vi "Part 1.vi"(11 "Input":string) -> (3 "Output":i64)   [LabVIEW 2021]
uses:
  8e0448e5-4d13-43f9-9dbd-05e23abb9177.vi
  <userlib>/_OpenG.lib/string/string.llb/Convert EOLs (String)__ogtk.vi
panel:
  out "array":string[](array[string])
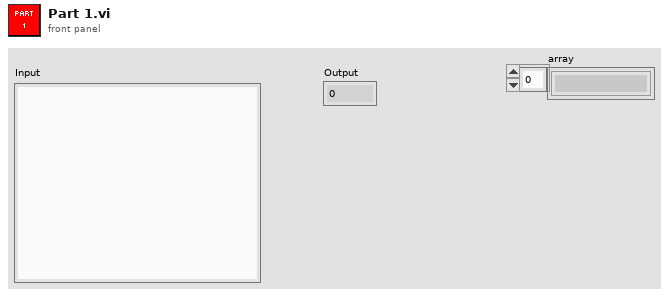
[diagram p1: front panel]
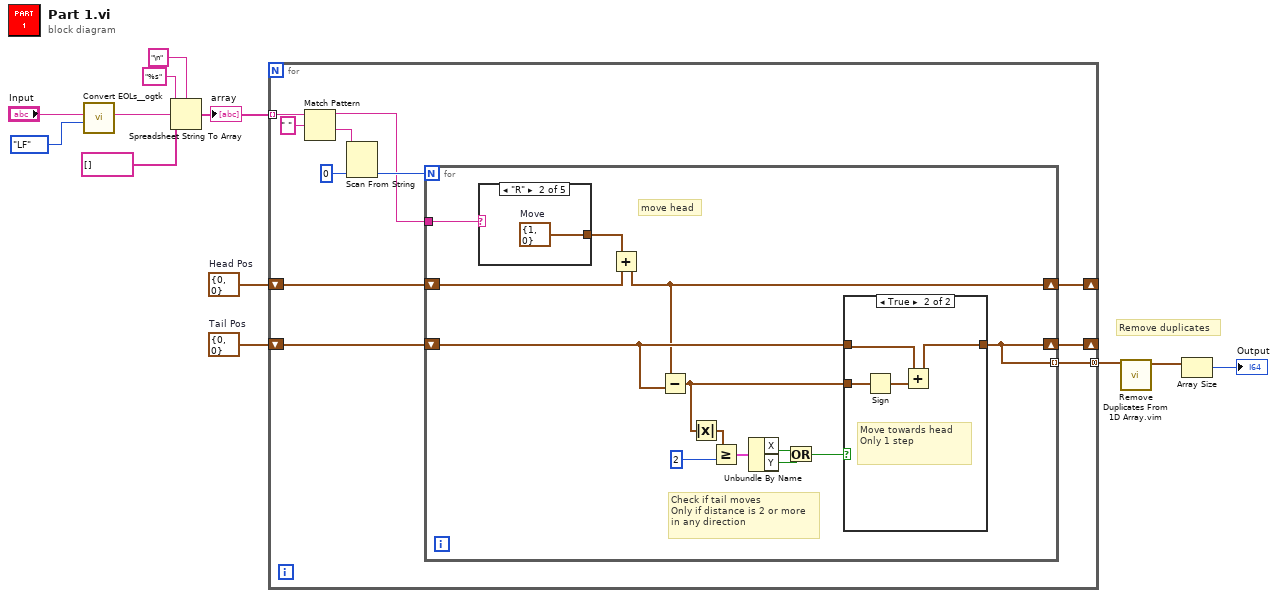
[diagram p0: block diagram]
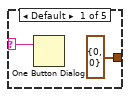
[diagram p3: hidden frame]
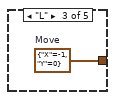
[diagram p4: hidden frame]
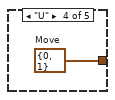
[diagram p5: hidden frame]
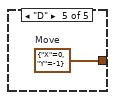
[diagram p6: hidden frame]
diagram:
  w4 = cluster{"X":i32, "Y":i32} {"X"=0, "Y"=0}  # Tail Pos
  w5 = cluster{"X":i32, "Y":i32} {"X"=0, "Y"=0}  # Head Pos
  # "Remove duplicates"
  n1 = call-poly <userlib>:"Convert EOLs__ogtk.vi"("Convert to:"=enum16{"CR", "LF", "CRLF"}."LF", "String in"="Input") -> ("String out"=w8:string)  [unwired: 9 in]
  n2 = Spreadsheet String To Array(delimiter (Tab)="\n", format string="%s", spreadsheet string=w8, array type (2D Dbl)=string[] []) -> (array=w6:string[])
  "array" <- w6
  n3 = for {
    tunnel: w6 -> [w23] mode=indexing
    shift-right: [w16] -> _
    shift-left: w5 -> [w18]
    shift-right: [w14] -> _
    shift-left: w4 -> [w17]
    tunnel: [w13] -> w3 mode=concatenating
    n4 = Match Pattern(string=w23, regular expression=" ") -> (before substring=w15:string, after substring=w21:string)  [unwired: 1 in, 2 out]
    n5 = Scan From String(input string=w21, default 1=0) -> (output 1=w19:i32)  [unwired: 3 in, 3 out]
    n6 = for {
      N: w19 -> [_]
      shift-right: [w25] -> w16
      shift-left: w18 -> [w35]
      shift-right: [w24] -> w14
      shift-left: w17 -> [w27]
      tunnel: w15 -> [w36]
      tunnel: [w24] -> w13 mode=indexing
      # "Check if tail moves\nOnly if distance is 2 or more\nin any direction"
      # "move head"
      n7 = case shown="\"R\"" w36 {
        selector: w36 -> [w43 _ _ _ _]
        tunnel: [cluster{"X":i32, "Y":i32} {"X"=0, "Y"=0} ("Move") w44 w45 w46 w47] -> w34
        frame Default {
          n8 = One Button Dialog(message=w43) -> ()  [unwired: 1 in, 1 out]
        }
        frame "R" {
          w44 = cluster{"X":i32, "Y":i32} {"X"=1, "Y"=0}  # Move
        }
        frame "L" {
          w45 = cluster{"X":i32, "Y":i32} {"X"=-1, "Y"=0}  # Move
        }
        frame "U" {
          w46 = cluster{"X":i32, "Y":i32} {"X"=0, "Y"=1}  # Move
        }
        frame "D" {
          w47 = cluster{"X":i32, "Y":i32} {"X"=0, "Y"=-1}  # Move
        }
      }
      n9 = Add(x=w34, y=w35) -> (x+y=w25:cluster{"X":i32, "Y":i32})
      n10 = Subtract(x=w25, y=w27) -> (x-y=w26:cluster{"X":i32, "Y":i32})
      n11 = Absolute Value(x=w26) -> (abs(x)=w29:cluster{"X":i32, "Y":i32})
      n12 = Greater Or Equal?(x=w29, y=2) -> (x >= y?=w32:cluster{"X":bool, "Y":bool})
      n13 = Unbundle By Name(w32) -> ("X"=w31:bool, "Y"=w30:bool)
      n14 = Or(x=w31, y=w30) -> (x .or. y?=w28:bool)
      n15 = case shown="True" w28 {
        tunnel: w27 -> [w37 w39]
        tunnel: [w37 w38] -> w24
        tunnel: w26 -> [_ w41]
        frame False {
        }
        frame True {
          # "Move towards head\nOnly 1 step"
          n16 = Sign(1:w41) -> (0:w40:cluster{"X":i32, "Y":i32})
          n17 = Add(x=w39, y=w40) -> (x+y=w38:cluster{"X":i32, "Y":i32})
        }
      }
    }
  }
  n18 = call "Remove Duplicates From 1D Array.vim"("array"=w3) -> ("array with duplicates removed"=w2:cluster{"X":i32, "Y":i32}[])  [unwired: 10 in]
  n19 = Array Size(array=w2) -> (size(s)=→"Output":i32)
